vi "五参数水样测试.vi"(11 "启动参数":T1={"测量模式"=enum."水样测试", "数据标记表"="N", "测量时间"=3.0}) -> ()   [LabVIEW 2016, in "斯坦道仪器.lvlib"]
uses:
  PLC/PLC.lvlib
panel:
  out "枚举":T2(ring)
  out "状态":string
  out "数值":i32
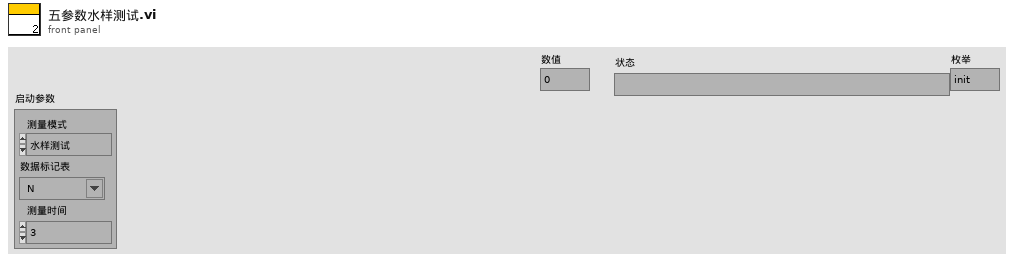
[diagram p1: front panel]
types:
  T1 = cluster{"测量模式":enum16{"待机", "水样测试", "标样核查", "零点核查", "跨度核查", "空白测试", "平行样测试", "加标回收", "空白校准", "标样校准", "初始化（清洗）"}, "数据标记表":string, "测量时间":dbl}
  T2 = enum16{"init", "开机", "启动测量", "读取测量值", "存储数据", "关闭测量", "关机", "结束"}
  T3 = cluster{"时间标识":timestamp, "设备":string, "日志信息":string, "流程参数":string}
  T4 = enum16{"待机", "水样测试", "标样核查", "零点核查", "跨度核查", "空白测试", "平行样测试", "加标回收", "空白校准", "标样校准", "初始化（清洗）"}
  T5 = cluster{"水温":dbl, "pH":dbl, "DO":dbl, "Cond":dbl, "Turb":dbl, "叶绿素":dbl, "藻密度":dbl, "蓝绿藻":dbl, "ORP":dbl, "NH3N":dbl}
  T6 = cluster{"数据标记表":string, "测量模式":enum16{"待机", "水样测试", "标样核查", "零点核查", "跨度核查", "空白测试", "平行样测试", "加标回收", "空白校准", "标样校准", "初始化（清洗）"}, "database":string}
  T7 = cluster{"因子编码":string, "单位":string, "标样参考值":sgl, "水样数据时间":timestamp, "水样实测值":sgl, "水样数据标识":string, "K":sgl, "B":sgl, "T":sgl, "H":sgl, "水深":sgl, "探头温度":sgl}
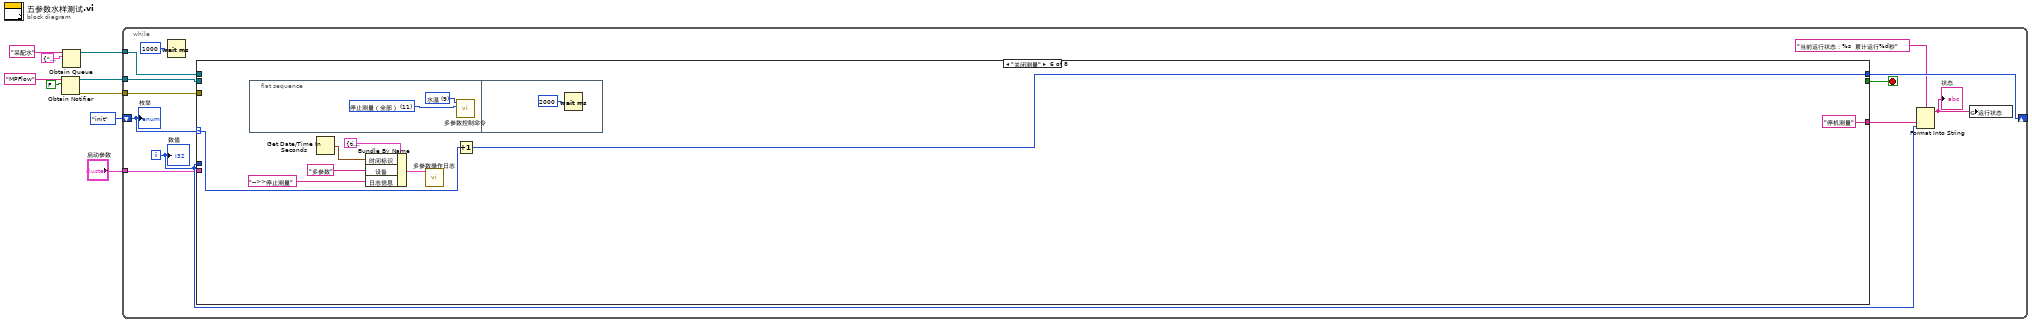
[diagram p0: block diagram]
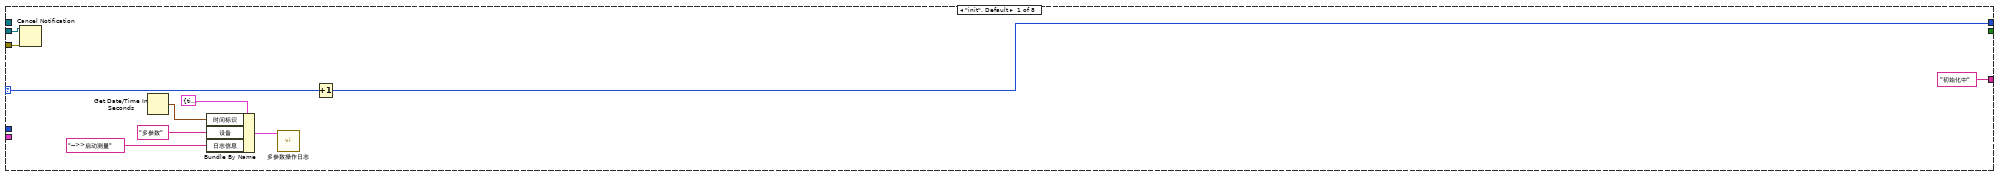
[diagram p2: hidden frame]
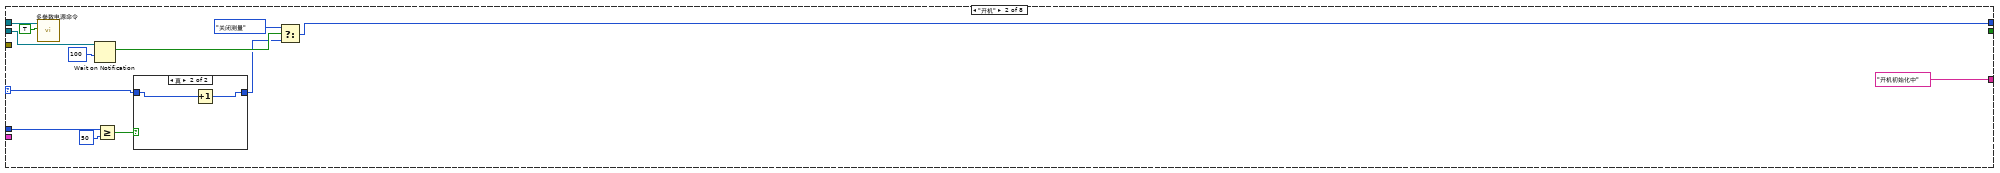
[diagram p3: hidden frame]
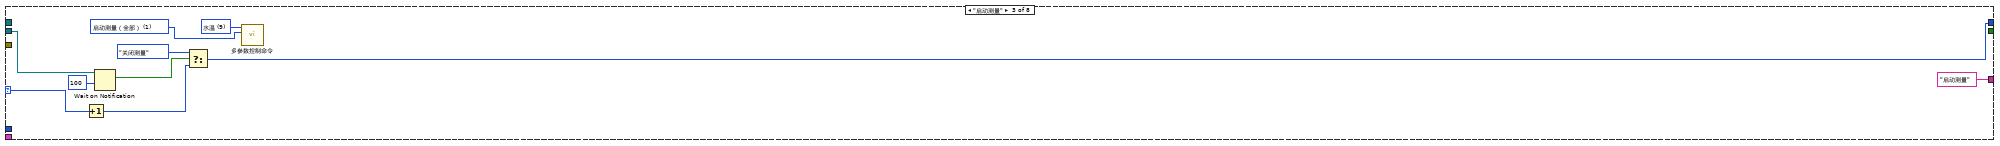
[diagram p5: hidden frame]
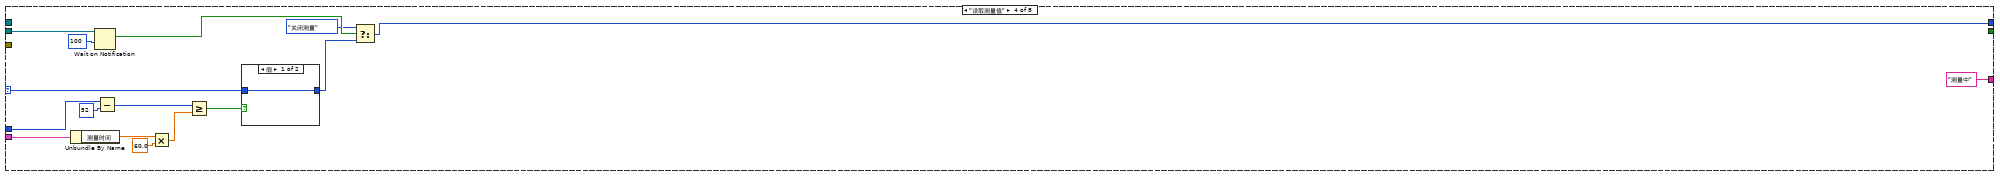
[diagram p6: hidden frame]
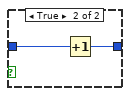
[diagram p7: hidden frame]
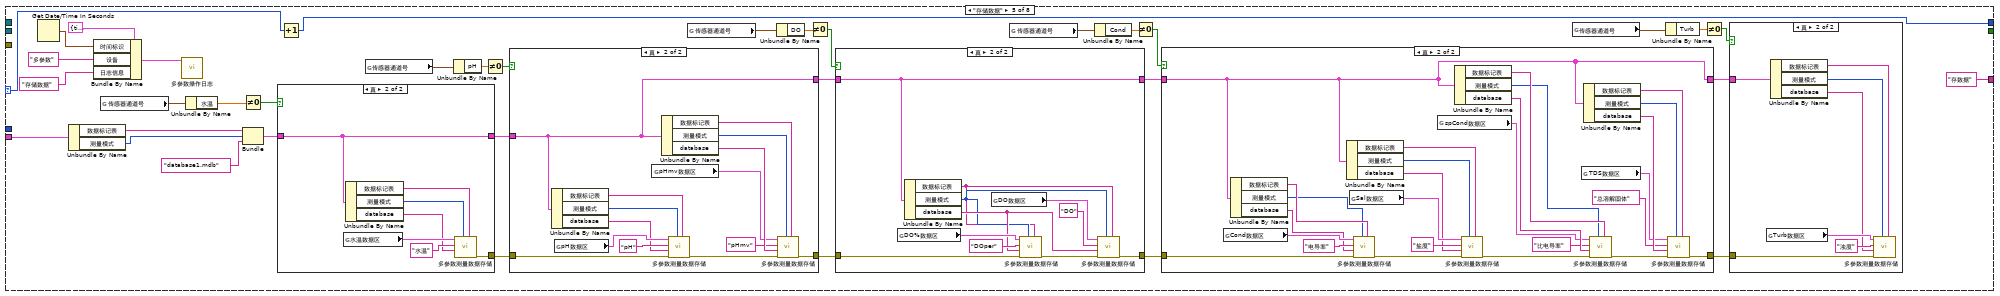
[diagram p8: hidden frame]
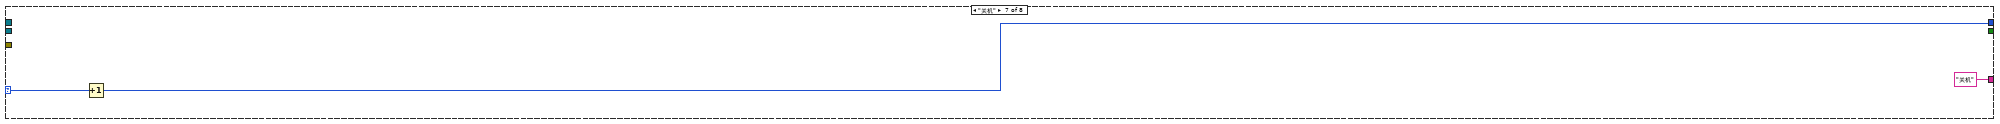
[diagram p14: hidden frame]
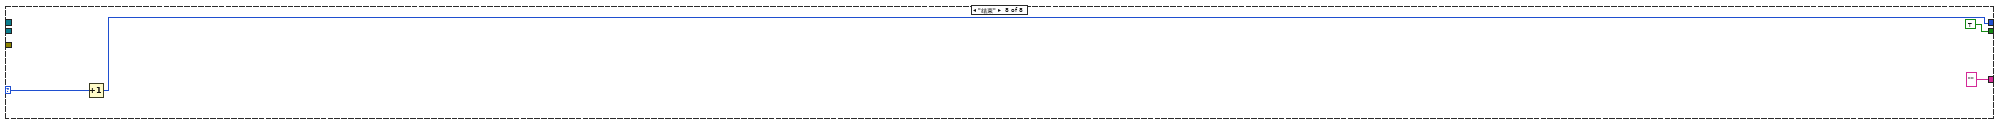
[diagram p15: hidden frame]
diagram:
  n1 = Obtain Notifier(name (unnamed)="MPFlow" ("名称（未命名）"), notification data type=FALSE) -> (notifier out=w6:refnum<notifier>, error out=w5:errorcluster)  [unwired: 2 in, 1 out]
  n2 = Obtain Queue(name (unnamed)="采配水" ("名称（未命名）"), element data type=cluster{"命令":string, "数据":variant} {"命令"="", "数据"=variant}) -> (queue out=w1:refnum<queue>)  [unwired: 3 in, 2 out]
  n3 = while {
    shift-right: [w17] -> _
    shift-left: T2."init" ("枚举") -> [w21]
    tunnel: w6 -> [w19]
    tunnel: w5 -> [w18]
    tunnel: "启动参数" -> [w11]
    tunnel: w1 -> [w10]
    i -> [w13]
    stop <- w20 stop-if-true
    n4 = Wait (ms)(milliseconds to wait=u32 1000 ("等待时间（毫秒）")) -> ()  [unwired: 1 out]
    n5 = case shown="\"关闭测量\"" w21 {
      selector: w21 -> [w29 w44 w57 w73 w112 w189 w195 w198]
      tunnel: [_ _ _ _ _ _ _ TRUE] -> w20
      tunnel: w19 -> [w31 w39 w56 w70 _ _ _ _]
      tunnel: w18 -> [w30 _ _ _ _ _ _ _]
      tunnel: [w28 w37 w53 w68 w111 w188 w194 w197] -> w17
      tunnel: w13 -> [_ w43 _ w60 _ _ _ _]
      tunnel: ["初始化中" ("状态") "开机初始化中" ("状态") "启动测量" ("状态") "测量中" ("状态") "存数据" ("状态") "停机测量" ("状态") "关机" ("状态") "" ("状态")] -> w14
      tunnel: w11 -> [_ _ _ w64 w109 _ _ _]
      tunnel: w10 -> [_ w33 _ _ _ _ _ _]
      frame "init", Default {
        n6 = Cancel Notification(0:w31, 3:w30) -> ()  [unwired: 3 out]
        n7 = Get Date/Time In Seconds() -> (seconds since 1Jan1904=w25:timestamp)
        n8 = Bundle By Name(cluster=T3 {"时间标识"=timestamp(0 s since 1904-01-01), "设备"="", "日志信息"="", "流程参数"=""} ("data in"), "时间标识"=w25, "设备"="多参数", "日志信息"="-->>启动测量") -> (w24:T3)
        n9 = call "多参数操作日志.vi"("data in"=w24) -> ()  [unwired: 10 in, 1 out]
        n10 = Increment(x=w29) -> (x+1=w28:T2)
      }
      frame "开机" {
        n11 = call "多参数电源命令.vi"("通电/断电"=TRUE, "队列"=w33) -> ()  [unwired: 9 in, 1 out]
        n12 = Wait on Notification(notifier=w39, timeout in ms (-1)=100 ("超时毫秒(-1)")) -> (notification=w40:bool)  [unwired: 2 in, 3 out]
        n13 = Greater Or Equal?(x=w43, y=50) -> (x >= y?=w41:bool)
        n14 = case shown="真" w41 {
          tunnel: w44 -> [w45 w47]
          tunnel: [w45 w46] -> w38
          frame False {
          }
          frame True {
            n15 = Increment(x=w47) -> (x+1=w46:T2)
          }
        }
        n16 = Select(t=T2."关闭测量" ("枚举"), s=w40, f=w38) -> (s? t:f=w37:T2)
      }
      frame "启动测量" {
        w48 = u16 1 items=["启动测量（全部）"=1, "初始化（清洗）"=10, "停止测量（全部）"=11, "校时"=13, "启动测量（单个传感器）"=19, "停止测量（单个传感器）"=20] ("控制命令")
        w49 = u16 9 items=["氨氮"=3, "水温"=9, "pH值"=10, "溶解氧"=11, "电导率"=12, "浊度"=13, "叶绿素a"=14, "藻密度"=15, "蓝绿藻"=16, "氧化还原电位"=17, "溶解氧%"=18, "盐度"=19] ("站号")
        n17 = Increment(x=w57) -> (x+1=w54:T2)
        n18 = Wait on Notification(notifier=w56, timeout in ms (-1)=100 ("超时毫秒(-1)")) -> (notification=w55:bool)  [unwired: 2 in, 3 out]
        n19 = Select(t=T2."关闭测量" ("枚举"), s=w55, f=w54) -> (s? t:f=w53:T2)
        n20 = call "多参数控制命令.vi"("控制命令"=w48, "站号"=w49) -> ()  [unwired: 9 in, 1 out]
      }
      frame "读取测量值" {
        n21 = Unbundle By Name(w64) -> ("测量时间"=w63:dbl)
        n22 = Wait on Notification(notifier=w70, timeout in ms (-1)=100 ("超时毫秒(-1)")) -> (notification=w71:bool)  [unwired: 2 in, 3 out]
        n23 = Subtract(x=w60, y=52) -> (x-y=w59:i32)
        n24 = Multiply(x=w63, y=60.0) -> (x*y=w61:dbl)
        n25 = Greater Or Equal?(x=w59, y=w61) -> (x >= y?=w72:bool)
        n26 = case shown="假" w72 {
          tunnel: w73 -> [w74 w76]
          tunnel: [w74 w75] -> w69
          frame False {
          }
          frame True {
            n27 = Increment(x=w76) -> (x+1=w75:T2)
          }
        }
        n28 = Select(t=T2."关闭测量" ("枚举"), s=w71, f=w69) -> (s? t:f=w68:T2)
      }
      frame "存储数据" {
        n29 = Get Date/Time In Seconds() -> (seconds since 1Jan1904=w80:timestamp)
        n30 = Unbundle By Name(w109) -> ("数据标记表"=w88:string, "测量模式"=w87:T4)
        n31 = Bundle By Name(cluster=T3 {"时间标识"=timestamp(0 s since 1904-01-01), "设备"="", "日志信息"="", "流程参数"=""} ("data in"), "时间标识"=w80, "设备"="多参数", "日志信息"="存储数据") -> (w79:T3)
        n32 = global read "多参数全局变量.vi" "传感器通道号"() -> (w104:T5)
        n33 = call "多参数操作日志.vi"("data in"=w79) -> ()  [unwired: 10 in, 1 out]
        n34 = Unbundle By Name(w104) -> ("水温"=w103:dbl)
        n35 = Not Equal To 0?(x=w103) -> (x != 0?=w102:bool)
        n36 = Bundle("数据标记表"=w88, "测量模式"=w87, "database"="database1.mdb") -> (w86:T6)  [unwired: 1 in]
        n37 = case shown="真" w102 {
          tunnel: [_ w179] -> w108
          tunnel: w86 -> [w174 w178]
          tunnel: [w174 w178] -> w85
          frame False {
          }
          frame True {
            n38 = global read "多参数全局变量.vi" "水温数据区"() -> (w181:T7)
            n39 = Unbundle By Name(w178) -> ("数据标记表"=w177:string, "测量模式"=w176:T4, "database"=w175:string)
            n40 = call "多参数测量数据存储.vi"("数据标记表"=w177, "测量模式"=w176, "database"=w175, "table输入"="水温", "data in"=w181) -> ("error out"=w179:errorcluster)  [unwired: 6 in]
          }
        }
        n41 = Increment(x=w112) -> (x+1=w111:T2)
        n42 = global read "多参数全局变量.vi" "传感器通道号"() -> (w97:T5)
        n43 = Unbundle By Name(w97) -> ("pH"=w96:dbl)
        n44 = Not Equal To 0?(x=w96) -> (x != 0?=w101:bool)
        n45 = case shown="真" w101 {
          tunnel: w108 -> [_ w173]
          tunnel: [_ w162] -> w107
          tunnel: w85 -> [w159 w167]
          tunnel: [w159 w167] -> w83
          frame False {
          }
          frame True {
            n46 = Unbundle By Name(w167) -> ("数据标记表"=w170:string, "测量模式"=w169:T4, "database"=w168:string)
            n47 = global read "多参数全局变量.vi" "pH数据区"() -> (w172:T7)
            n48 = global read "多参数全局变量.vi" "pHmv数据区"() -> (w161:T7)
            n49 = Unbundle By Name(w167) -> ("数据标记表"=w166:string, "测量模式"=w165:T4, "database"=w164:string)
            n50 = call "多参数测量数据存储.vi"("数据标记表"=w170, "测量模式"=w169, "error in (no error)"=w173, "database"=w168, "table输入"="pH", "data in"=w172) -> ("error out"=w163:errorcluster)  [unwired: 5 in]
            n51 = call "多参数测量数据存储.vi"("数据标记表"=w166, "测量模式"=w165, "error in (no error)"=w163, "database"=w164, "table输入"="pHmv", "data in"=w161) -> ("error out"=w162:errorcluster)  [unwired: 5 in]
          }
        }
        n52 = global read "多参数全局变量.vi" "传感器通道号"() -> (w95:T5)
        n53 = Unbundle By Name(w95) -> ("DO"=w94:dbl)
        n54 = Not Equal To 0?(x=w94) -> (x != 0?=w100:bool)
        n55 = case shown="真" w100 {
          tunnel: w107 -> [_ w158]
          tunnel: [_ w154] -> w106
          tunnel: [w147 w151] -> w84
          tunnel: w83 -> [w147 w151]
          frame False {
          }
          frame True {
            n56 = global read "多参数全局变量.vi" "DO%数据区"() -> (w153:T7)
            n57 = Unbundle By Name(w151) -> ("数据标记表"=w148:string, "测量模式"=w149:T4, "database"=w150:string)
            n58 = global read "多参数全局变量.vi" "DO数据区"() -> (w155:T7)
            n59 = call "多参数测量数据存储.vi"("数据标记表"=w148, "测量模式"=w149, "error in (no error)"=w158, "database"=w150, "table输入"="DOper", "data in"=w153) -> ("error out"=w157:errorcluster)  [unwired: 5 in]
            n60 = call "多参数测量数据存储.vi"("数据标记表"=w148, "测量模式"=w149, "error in (no error)"=w157, "database"=w150, "table输入"="DO", "data in"=w155) -> ("error out"=w154:errorcluster)  [unwired: 5 in]
          }
        }
        n61 = global read "多参数全局变量.vi" "传感器通道号"() -> (w93:T5)
        n62 = Unbundle By Name(w93) -> ("Cond"=w92:dbl)
        n63 = Not Equal To 0?(x=w92) -> (x != 0?=w99:bool)
        n64 = case shown="真" w99 {
          tunnel: w106 -> [_ w144]
          tunnel: [_ w125] -> w105
          tunnel: w84 -> [w120 w134]
          tunnel: [w120 w134] -> w82
          frame False {
          }
          frame True {
            n65 = global read "多参数全局变量.vi" "Cond数据区"() -> (w146:T7)
            n66 = Unbundle By Name(w134) -> ("数据标记表"=w139:string, "测量模式"=w138:T4, "database"=w140:string)
            n67 = Unbundle By Name(w134) -> ("数据标记表"=w137:string, "测量模式"=w136:T4, "database"=w135:string)
            n68 = global read "多参数全局变量.vi" "Sal数据区"() -> (w142:T7)
            n69 = call "多参数测量数据存储.vi"("数据标记表"=w139, "测量模式"=w138, "error in (no error)"=w144, "database"=w140, "table输入"="电导率", "data in"=w146) -> ("error out"=w143:errorcluster)  [unwired: 5 in]
            n70 = global read "多参数全局变量.vi" "spCond数据区"() -> (w124:T7)
            n71 = Unbundle By Name(w134) -> ("数据标记表"=w133:string, "测量模式"=w132:T4, "database"=w131:string)
            n72 = call "多参数测量数据存储.vi"("数据标记表"=w137, "测量模式"=w136, "error in (no error)"=w143, "database"=w135, "table输入"="盐度", "data in"=w142) -> ("error out"=w130:errorcluster)  [unwired: 5 in]
            n73 = global read "多参数全局变量.vi" "TDS数据区"() -> (w123:T7)
            n74 = Unbundle By Name(w134) -> ("数据标记表"=w126:string, "测量模式"=w127:T4, "database"=w128:string)
            n75 = call "多参数测量数据存储.vi"("数据标记表"=w133, "测量模式"=w132, "error in (no error)"=w130, "database"=w131, "table输入"="比电导率", "data in"=w124) -> ("error out"=w129:errorcluster)  [unwired: 5 in]
            n76 = call "多参数测量数据存储.vi"("数据标记表"=w126, "测量模式"=w127, "error in (no error)"=w129, "database"=w128, "table输入"="总溶解固体", "data in"=w123) -> ("error out"=w125:errorcluster)  [unwired: 5 in]
          }
        }
        n77 = global read "多参数全局变量.vi" "传感器通道号"() -> (w91:T5)
        n78 = Unbundle By Name(w91) -> ("Turb"=w90:dbl)
        n79 = Not Equal To 0?(x=w90) -> (x != 0?=w98:bool)
        n80 = case shown="真" w98 {
          tunnel: w105 -> [_ w119]
          tunnel: w82 -> [_ w116]
          frame False {
          }
          frame True {
            n81 = global read "多参数全局变量.vi" "Turb数据区"() -> (w118:T7)
            n82 = Unbundle By Name(w116) -> ("数据标记表"=w113:string, "测量模式"=w114:T4, "database"=w115:string)
            n83 = call "多参数测量数据存储.vi"("数据标记表"=w113, "测量模式"=w114, "error in (no error)"=w119, "database"=w115, "table输入"="浊度", "data in"=w118) -> ()  [unwired: 5 in, 1 out]
          }
        }
      }
      frame "关闭测量" {
        n84 = flat-sequence {
          frame #0 {
            w190 = u16 11 items=["启动测量（全部）"=1, "初始化（清洗）"=10, "停止测量（全部）"=11, "校时"=13, "启动测量（单个传感器）"=19, "停止测量（单个传感器）"=20] ("控制命令")
            w191 = u16 9 items=["氨氮"=3, "水温"=9, "pH值"=10, "溶解氧"=11, "电导率"=12, "浊度"=13, "叶绿素a"=14, "藻密度"=15, "蓝绿藻"=16, "氧化还原电位"=17, "溶解氧%"=18, "盐度"=19] ("站号")
            n85 = call "多参数控制命令.vi"("控制命令"=w190, "站号"=w191) -> ()  [unwired: 9 in, 1 out]
          }
          frame #1 {
            n86 = Wait (ms)(milliseconds to wait=u32 2000 ("等待时间（毫秒）")) -> ()  [unwired: 1 out]
          }
        }
        n87 = Get Date/Time In Seconds() -> (seconds since 1Jan1904=w185:timestamp)
        n88 = Bundle By Name(cluster=T3 {"时间标识"=timestamp(0 s since 1904-01-01), "设备"="", "日志信息"="", "流程参数"=""} ("data in"), "时间标识"=w185, "设备"="多参数", "日志信息"="-->>停止测量") -> (w184:T3)
        n89 = call "多参数操作日志.vi"("data in"=w184) -> ()  [unwired: 10 in, 1 out]
        n90 = Increment(x=w189) -> (x+1=w188:T2)
      }
      frame "关机" {
        n91 = Increment(x=w195) -> (x+1=w194:T2)
      }
      frame "结束" {
        n92 = Increment(x=w198) -> (x+1=w197:T2)
      }
    }
    n93 = Format Into String(format string="当前运行状态：%s  累计运行%d秒" ("格式字符串"), w14, w13) -> (resulting string=w12:string)  [unwired: 2 in, 1 out]
    "状态" <- w12
    n94 = global write "多参数全局变量.vi" "运行状态"(w12) -> ()
    "数值" <- w13
    "枚举" <- w21
  }
